vi "InitPort.vi"(6 "timeout":dbl, 8 "error in (no error)":errorcluster, 9 "Baud":u32=115200, 10 "Port":string, 11 "Python":T1) -> (0 "error out":errorcluster, 2 "Console":string, 3 "Python out":T1)   [LabVIEW 2022 SP3]
uses:
  PythonCtrl.ctl
  Processors.ctl
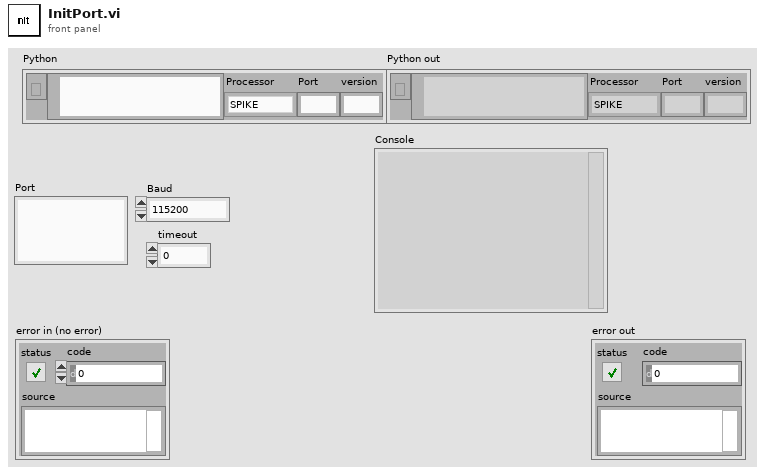
[diagram p1: front panel]
types:
  T1 = typedef "PythonCtrl.ctl" = cluster{"session":refnum<k35>, "PyPath":path, "Processor":T2, "Port":string, "version":string}
  T2 = typedef "Processors.ctl" = enum16{"SPIKE", "Pi", "Pi_ssh", "OpenMV", "Dunio"}
  T3 = cluster{"IP Address":string, "Username":string, "password":string}
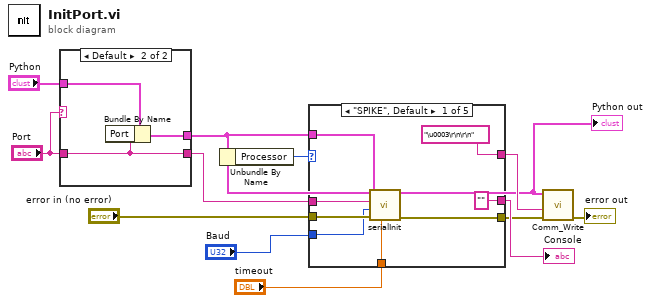
[diagram p0: block diagram]
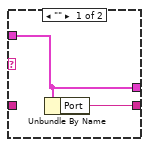
[diagram p2: hidden frame]
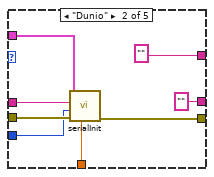
[diagram p3: hidden frame]
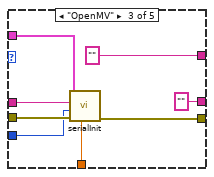
[diagram p4: hidden frame]
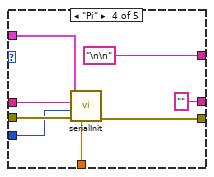
[diagram p5: hidden frame]
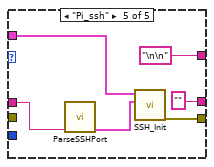
[diagram p6: hidden frame]
diagram:
  n1 = case shown="Default" "Port" {
    tunnel: "Python" -> [w14 w17]
    tunnel: [w14 w16] -> w3
    tunnel: "Port" -> [_ w15]
    tunnel: [w13 w15] -> w1
    frame "" {
      n2 = Unbundle By Name(w14) -> ("Port"=w13:string)
    }
    frame Default {
      n3 = Bundle By Name(cluster=w17, "Port"=w15) -> (w16:T1)
    }
  }
  "Python out" <- w3
  n4 = Unbundle By Name(w3) -> ("Processor"=w12:T2)
  n5 = case shown="\"SPIKE\", Default" w12 {
    tunnel: ["\u0003\r\n\r\n" ("function name") "" ("function name") "" ("function name") "\n\n" ("function name") "\n\n" ("function name")] -> w8
    tunnel: "error in (no error)" -> [w24 w32 w40 w48 _]
    tunnel: w1 -> [w23 w31 w39 w47 w51]
    tunnel: w3 -> [w22 w30 w38 w46 w54]
    tunnel: [w21 w29 w37 w45 w53] -> w6
    tunnel: "Baud" -> [w20 w28 w36 w44 _]
    tunnel: "timeout" -> [w19 w27 w35 w43 _]
    tunnel: ["" ("function name") "" ("function name") "" ("function name") "" ("function name") "" ("function name")] -> w7
    frame "SPIKE", Default {
      n6 = call "serialInit.vi"("timeout"=w19, "error in (no error)"=w24, "Baud"=w20, "Port"=w23, "Python"=w22) -> ("error out"=w21:errorcluster)  [unwired: 4 in, 2 out]
    }
    frame "Dunio" {
      n7 = call "serialInit.vi"("timeout"=w27, "error in (no error)"=w32, "Baud"=w28, "Port"=w31, "Python"=w30) -> ("error out"=w29:errorcluster)  [unwired: 4 in, 2 out]
    }
    frame "OpenMV" {
      n8 = call "serialInit.vi"("timeout"=w35, "error in (no error)"=w40, "Baud"=w36, "Port"=w39, "Python"=w38) -> ("error out"=w37:errorcluster)  [unwired: 4 in, 2 out]
    }
    frame "Pi" {
      n9 = call "serialInit.vi"("timeout"=w43, "error in (no error)"=w48, "Baud"=w44, "Port"=w47, "Python"=w46) -> ("error out"=w45:errorcluster)  [unwired: 4 in, 2 out]
    }
    frame "Pi_ssh" {
      n10 = call "ParseSSHPort.vi"("String in"=w51) -> ("port"=w50:T3)  [unwired: 8 in, 2 out]
      n11 = call "SSH_Init.vi"("Raspberry Pi"=w50, "Python in"=w54) -> ("error out"=w53:errorcluster)  [unwired: 7 in, 2 out]
    }
  }
  "Console" <- w7
  n12 = call "Comm_Write.vi"("error in (no error)"=w6, "Text to write"=w8, "Python"=w3) -> ("error out"=→"error out":errorcluster)  [unwired: 7 in, 1 out]
